vi "Find_Potentially_Stat_Dots_In_Dot-Matrix-2.vi"(0 "[IN] Collecting array":dbl[](array[numeric]), 1 "Finish Position\n(Collecting arr)":i32, 2 "[IN] Possibly \nMoving Dots \n(Column)":dbl[](array[numeric]), 3 "[IN] Dot matrix":i16[](array[numeric]), 4 "Number\nof \"+1\"":i32) -> (5 "[OUT] Dot matrix":i16[](array[numeric]), 6 "Number of such\nassignments":i32)   [LabVIEW 2013]
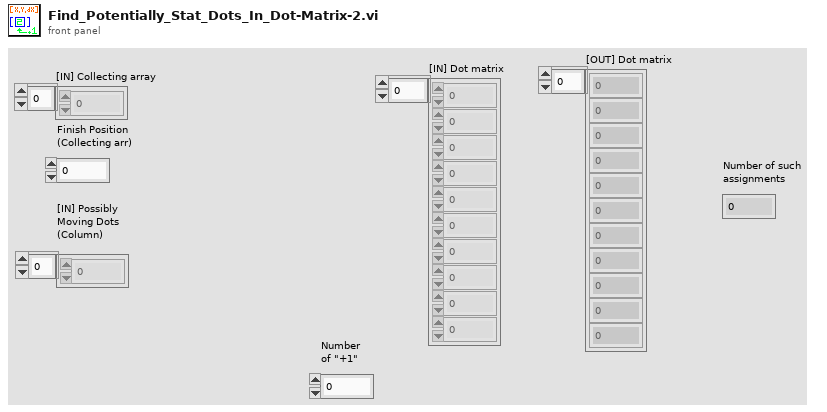
[diagram p1: front panel]
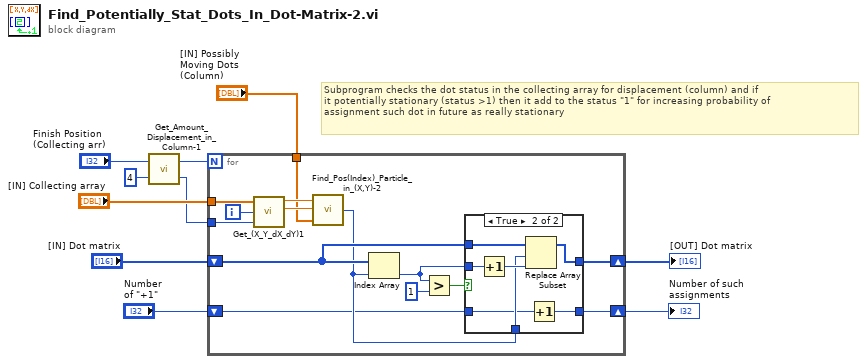
[diagram p0: block diagram]
diagram:
  # "Subprogram checks the dot status in the collecting array for displacement (column) and if\nit potentially stationary (status >1) then it add to the status \"1\" for increasing probability of \nassignment such dot in future as really stationary"
  n1 = call "Get_Amount_Displacement_in_Column-1.vi"("multiplier"=4 ("y"), "# Rows"="Finish Position\n(Collecting arr)") -> ("multiplier out"=w6:i32, "Displ amount"=w8:i32)
  n2 = for {
    N: w8 -> [_]
    tunnel: "[IN] Collecting array" -> [w24]
    tunnel: w6 -> [w22]
    tunnel: "[IN] Possibly \nMoving Dots \n(Column)" -> [w18]
    shift-right: [w13] -> w3
    shift-left: "[IN] Dot matrix" -> [w15]
    shift-right: [w11] -> w1
    shift-left: "Number\nof \"+1\"" -> [w12]
    i -> [w23]
    n3 = call "Get_(X_Y_dX_dY)1.vi"("(X,Y,dX,dY)"=w24, "index"=w23, "multiplier"=w22) -> ("X"=w21:dbl, "Y"=w20:dbl)  [unwired: 2 out]
    n4 = call "Find_Pos(Index)_Particle_in_(X,Y)-2.vi"("[X,Y] (n Frame)"=w18, "Y1"=w20, "X1"=w21) -> ("Index in (n) Frame"=w14:i32)
    n5 = Index Array(array=w15, index=w14) -> (element=w16:i16)
    n6 = Greater?(x=w16, y=i16 1) -> (0:w17:bool)
    n7 = case shown="True" w17 {
      tunnel: w16 -> [_ w33]
      tunnel: w15 -> [w26 w32]
      tunnel: w14 -> [_ w30]
      tunnel: [w26 w29] -> w13
      tunnel: w12 -> [w25 w28]
      tunnel: [w25 w27] -> w11
      frame False {
      }
      frame True {
        n8 = Increment(x=w33) -> (x+1=w31:i16)
        n9 = Replace Array Subset(array=w32, new element=w31, index=w30) -> (w29:i16[])
        n10 = Increment(x=w28) -> (x+1=w27:i32)
      }
    }
  }
  "[OUT] Dot matrix" <- w3
  "Number of such\nassignments" <- w1
